vi "sio close.vi"(10 "port":i32) -> (2 "function return":i32, 3 "port":i32)   [LabVIEW 2012, in "PCOMM.lvlib"]
doc: "int WINAPI sio_close(int port);"
uses:
  PCOMM.lvlib
  #001 2018-09-10/Data/PCOMM.DLL
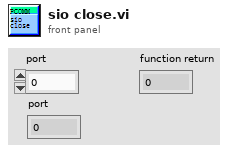
[diagram p1: front panel]
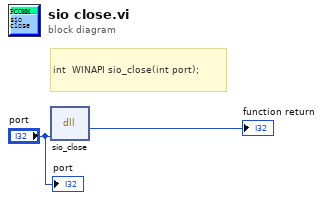
[diagram p0: block diagram]
diagram:
  # "int  WINAPI sio_close(int port);"
  n1 = dll-call lib="E:/ProJect/#008 ESDMonitor/#002 Labview/#001 2018-09-10/Data/PCOMM.*" fn="sio_close"("port"="port") -> (→"function return":i32)  [unwired: 4 in, 2 out]
  "port" <- "port"
